vi "Broadcast Map.vi"(8 "error in (no error)":errorcluster, 11 "Map Model in":refnum<class "Map Model.lvclass">) -> (0 "error out":errorcluster, 3 "Map Model out":refnum<class "Map Model.lvclass">)   [LabVIEW 2020, in "Map Model.lvlib" / "Map Model.lvclass"]
uses:
  Map Model.lvclass
  Map Model Messages/Abstract Map Msg/Abstract Map Msg.lvclass
  C:/Program Files/National Instruments/LabVIEW 2020/vi.lib/ActorFrameworkObserver/Data Message/Data Message.lvclass
  Map Model.lvclass/Map Model.ctl
  <vilib>/ActorFrameworkObserver/Actor Register/Actor Register.lvclass
panel:
  # "NOTICE -- YOU MUST LEAVE THIS NOTICE IN PLACE.\n\nCopyright (c) 2017, LIANG LIU Shawn.Liu.cn@gmail.com\nAll rights reserved.\n\nRedistribution and use in source and binary forms, with or without modification, are permitted provided that the following conditions are met:\n-Redistributions of source code must retain the above copyright notice, this list of conditions and the following disclaimer.\n-Redistributions in binary form must reproduce the above copyright notice, this list of conditions and the following disclaimer in the documentation and/or other materials provided with the distribution.\n-Neither the name of the eLp nor the names of its contributors may be used to endorse or promote products derived from this software without specific prior written permission.\n\nTHIS SOFTWARE IS PROVIDED BY THE COPYRIGHT HOLDERS AND CONTRIBUTORS \"AS IS\" AND ANY EXPRESS OR IMPLIED WARRANTIES, INCLUDING, BUT NOT LIMITED TO, THE IMPLIED WARRANTIES OF MERCHANTABILITY AND FITNESS FOR A PARTICULAR PURPOSE ARE DISCLAIMED. IN NO EVENT SHALL THE COPYRIGHT HOLDER OR CONTRIBUTORS BE LIABLE FOR ANY DIRECT, INDIRECT, INCIDENTAL, SPECIAL, EXEMPLARY, OR CONSEQUENTIAL DAMAGES (INCLUDING, BUT NOT LIMITED TO, PROCUREMENT OF SUBSTITUTE GOODS OR SERVICES; LOSS OF USE, DATA, OR PROFITS; OR BUSINESS INTERRUPTION) HOWEVER CAUSED AND ON ANY THEORY OF LIABILITY, WHETHER IN CONTRACT, STRICT LIABILITY, OR TORT (INCLUDING NEGLIGENCE OR OTHERWISE) ARISING IN ANY WAY OUT OF THE USE OF THIS SOFTWARE, EVEN IF ADVISED OF THE POSSIBILITY OF SUCH DAMAGE."
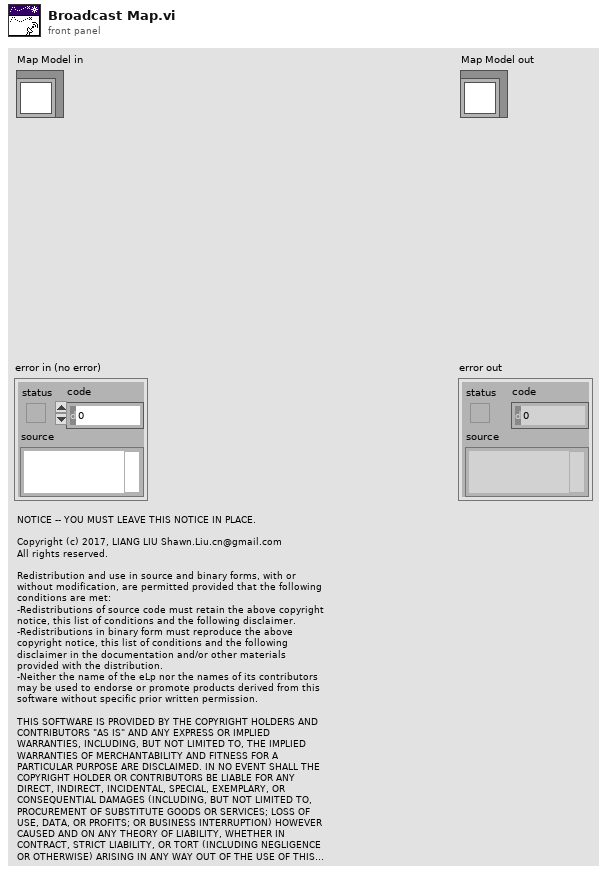
[diagram p1: front panel]
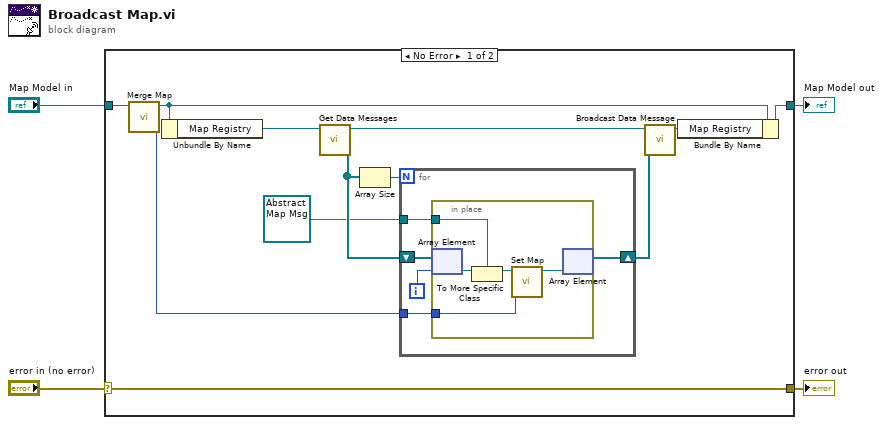
[diagram p0: block diagram]
diagram:
  n1 = case shown="No Error" "error in (no error)" {
    selector: "error in (no error)" -> [w14 w28]
    tunnel: "Map Model in" -> [w16 w27]
    tunnel: [w15 w27] -> w3
    tunnel: [w14 w28] -> w1
    frame No Error {
      n2 = call "Merge Map.vi"("Map Model in"=w16) -> ("Map"=w5:picture, "Map Model out"=w6:refnum<class "Map Model.lvclass">)  [unwired: 8 in, 1 out]
      n3 = Unbundle By Name(w6) -> ("Map Registry"=w13:refnum<class "Actor Register.lvclass">)
      n4 = call-dynamic "Get Data Messages.vi"("Actor Register in"=w13) -> ("Data Messages"=w10:refnum<class "Data Message.lvclass">[], "Actor Register out"=w12:refnum<class "Actor Register.lvclass">)  [unwired: 9 in]
      n5 = Array Size(array=w10) -> (size(s)=w8:i32)
      n6 = for {
        N: w8 -> [_]
        shift-right: [w19] -> w7
        shift-left: w10 -> [w21]
        tunnel: refnum<class "Abstract Map Msg.lvclass"> refnum ("Map Model.lvlib:Abstract Map Msg.lvclass") -> [w20]
        tunnel: w5 -> [w17]
        i -> [w18]
        n7 = in-place {
          in-place-border: w20 -> [w25]
          in-place-border: w17 -> [w22]
          n8 = in-place-array #1(w21, w18) -> (w26:refnum<class "Data Message.lvclass">)
          n9 = To More Specific Class(target class=w25, reference=w26) -> (specific class reference=w24:refnum<class "Abstract Map Msg.lvclass">)  [unwired: 1 in, 1 out]
          n10 = call "Set Map.vi"("Map"=w22, "Abstract Map Msg in"=w24) -> ("Abstract Map Msg out"=w23:refnum<class "Abstract Map Msg.lvclass">)  [unwired: 9 in]
          n11 = in-place-array #1(w23) -> (w19:refnum<class "Data Message.lvclass">[])  [unwired: 1 out]
        }
      }
      n12 = call <vilib>:"Broadcast Data Message.vi"("Data Messages"=w7, "Actor Register in"=w12) -> ("Actor Register out"=w11:refnum<class "Actor Register.lvclass">)  [unwired: 8 in, 1 out]
      n13 = Bundle By Name(cluster=w6, "Map Registry"=w11) -> (w15:refnum<class "Map Model.lvclass">)
    }
    frame Error {
    }
  }
  "error out" <- w1
  "Map Model out" <- w3
